vi "PT3_ImgHeaderToIntArray.vi"(11 "Image Header":T1) -> (3 "Array":i32[](array[numeric]))   [LabVIEW 2010]
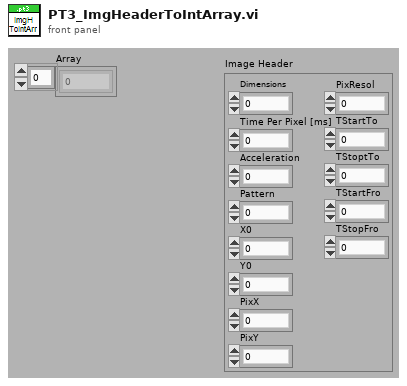
[diagram p1: front panel]
types:
  T1 = cluster{"Dimensions":i32, "Time Per Pixel [ms]":dbl, "Acceleration":i32, "Pattern":i32, "X0":sgl, "Y0":sgl, "PixX":i32, "PixY":i32, "PixResol":sgl, "TStartTo":sgl, "TStoptTo":sgl, "TStartFro":sgl, "TStopFro":sgl}
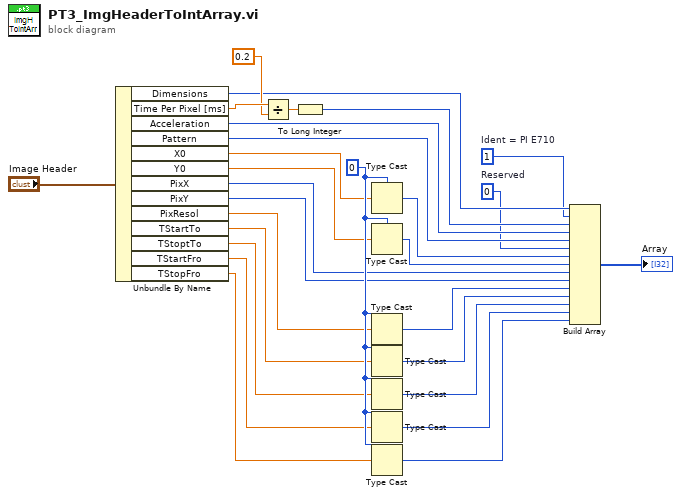
[diagram p0: block diagram]
diagram:
  w10 = 0  # Reserved
  w14 = 1  # Ident = PI E710
  w28 = 0
  n1 = Unbundle By Name("Image Header") -> ("Dimensions"=w15:i32, "Time Per Pixel [ms]"=w26:dbl, "Acceleration"=w12:i32, "Pattern"=w11:i32, "X0"=w23:sgl, "Y0"=w22:sgl, "PixX"=w6:i32, "PixY"=w7:i32, "PixResol"=w18:sgl, "TStartTo"=w17:sgl, "TStoptTo"=w20:sgl, "TStartFro"=w19:sgl, "TStopFro"=w21:sgl)
  n2 = Divide(x=w26, y=0.2) -> (x/y=w24:dbl)
  n3 = To Long Integer(number=w24) -> (32bit integer=w13:i32)
  n4 = Type Cast(type=w28, x=w23) -> (*(type *) &x=w8:i32)
  n5 = Type Cast(type=w28, x=w22) -> (*(type *) &x=w9:i32)
  n6 = Type Cast(type=w28, x=w18) -> (*(type *) &x=w4:i32)
  n7 = Type Cast(type=w28, x=w17) -> (*(type *) &x=w3:i32)
  n8 = Type Cast(type=w28, x=w20) -> (*(type *) &x=w2:i32)
  n9 = Type Cast(type=w28, x=w19) -> (*(type *) &x=w1:i32)
  n10 = Type Cast(type=w28, x=w21) -> (*(type *) &x=w5:i32)
  n11 = Build Array(w15, w14, w13, w12, w11, w10, w8, w9, w6, w7, w4, w3, w2, w1, w5) -> (→"Array":i32[])
